vi "Get Board Memory Size.vi"(8 "error in (no error)":errorcluster, 11 "GE 5565PIORC in":refnum<class "GE 5565PIORC.lvclass">) -> (0 "error out":errorcluster, 3 "GE 5565PIORC out":refnum<class "GE 5565PIORC.lvclass">)   [LabVIEW 2016, in "GE 5565PIORC.lvclass"]
uses:
  GE 5565PIORC.lvclass
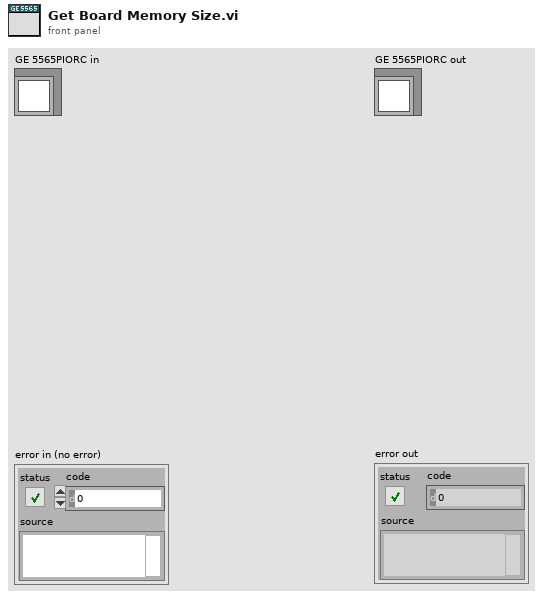
[diagram p1: front panel]
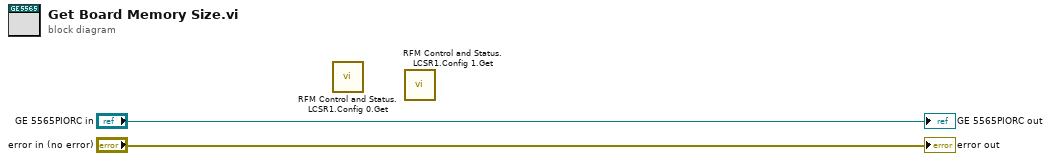
[diagram p0: block diagram]
diagram:
  n1 = call "RFM Control and Status.LCSR1.Config 0.Get.vi"() -> ()  [unwired: 9 in, 3 out]
  n2 = call "RFM Control and Status.LCSR1.Config 1.Get.vi"() -> ()  [unwired: 9 in, 3 out]
  "error out" <- "error in (no error)"
  "GE 5565PIORC out" <- "GE 5565PIORC in"
